vi "main_test.vi"() -> ()   [LabVIEW 2017]
panel:
  out "Locking ratio [%]":dbl
  in  "Excel data":path
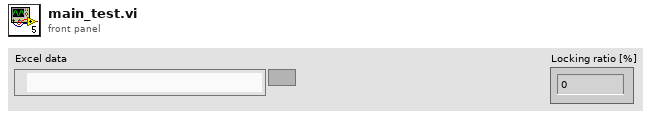
[diagram p1: front panel]
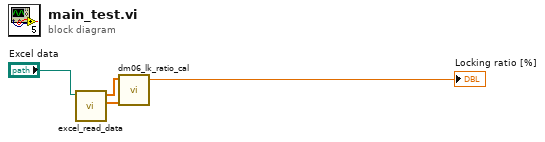
[diagram p0: block diagram]
diagram:
  n1 = call "excel_read_data.vi"("Excel data"="Excel data") -> ("wv_length_weight"=w2:dbl[], "wv_length_data"=w3:dbl[])  [unwired: 8 in, 1 out]
  n2 = call "dm06_lk_ratio_cal.vi"("Signal power input"=w2, "Wavelength_input"=w3) -> ("Locking ratio [%]"=→"Locking ratio [%]":dbl)  [unwired: 9 in]
